vi "Write configuration.vi"(8 "error in (no error)":errorcluster, 11 "Autofocus in":refnum<class "Autofocus.lvclass">) -> (0 "error out":errorcluster, 3 "Autofocus out":refnum<class "Autofocus.lvclass">)   [LabVIEW 2012, in "Autofocus.lvclass"]
doc: "Writes the configuration cluster into the configuration file. Configuration file is XML-based. It's name is <component ID>.xml"
uses:
  Autofocus.lvclass
  <vilib>/Distrio/Murmex/Murmex/Murmex.lvclass
  Autofocus.lvclass/Autofocus.ctl
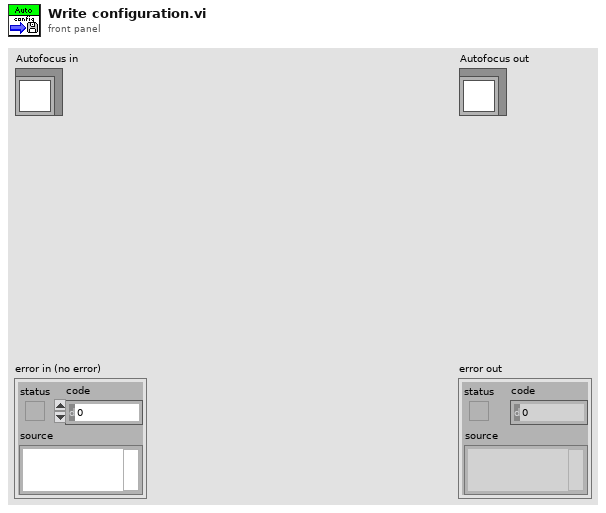
[diagram p1: front panel]
types:
  T1 = typedef "Autofocus.lvclass/configuration cluster.ctl" = cluster{"Numeric":dbl}
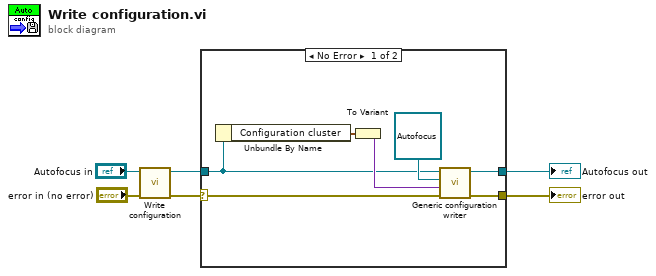
[diagram p0: block diagram]
diagram:
  n1 = call-parent "Write configuration.vi"("error in (no error)"="error in (no error)", "Murmex in"="Autofocus in") -> ("error out"=w4:errorcluster, "Murmex out"=w3:refnum<class "Autofocus.lvclass">)  [unwired: 8 in]
  n2 = case shown="No Error" w4 {
    selector: w4 -> [w12 w14]
    tunnel: w3 -> [w8 w15]
    tunnel: [w11 w14] -> w2
    tunnel: [w10 w15] -> w1
    frame No Error {
      n3 = Unbundle By Name(w8) -> ("Configuration cluster"=w7:T1)
      n4 = To Variant(anything=w7) -> (Variant=w9:variant)
      n5 = call <vilib>:"Generic configuration writer.vi"("error in (no error)"=w12, "configuration"=w9, "inheritance level"=refnum<class "Autofocus.lvclass"> refnum ("Autofocus.lvclass"), "MurmexBase in"=w8) -> ("error out"=w11:errorcluster, "MurmexBase out"=w10:refnum<class "Autofocus.lvclass">)  [unwired: 6 in]
    }
    frame Error {
    }
  }
  "error out" <- w2
  "Autofocus out" <- w1
